vi "comm_Write_ip.vi"() -> ()   [LabVIEW 2014]
panel:
  in  "Indicator":bool
  in  "stop":bool
  # "BOMET TEST COMUNICATION WRITE"
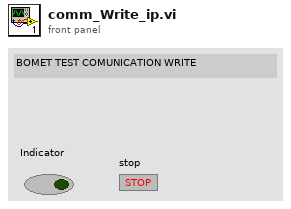
[diagram p1: front panel]
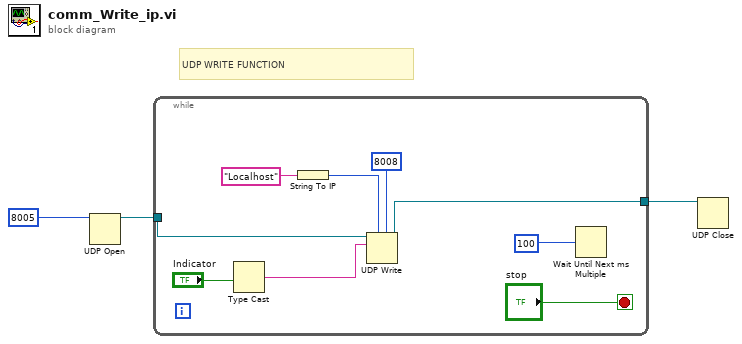
[diagram p0: block diagram]
diagram:
  # "UDP WRITE FUNCTION"
  n1 = UDP Open(11:u16 8005 ("port")) -> (port=w2:refnum<k16>)  [unwired: 4 in, 2 out]
  n2 = while {
    tunnel: w2 -> [w12]
    tunnel: [w11] -> w1
    stop <- "stop" stop-if-true
    n3 = Type Cast(x="Indicator") -> (*(type *) &x=w6:string)  [unwired: 1 in]
    n4 = String To IP(1:"Localhost" ("name")) -> (0:w9:u32)
    n5 = UDP Write(address=w9, port or service name=u16 8008, connection ID=w12, data in=w6) -> (3:w11:refnum<k16>)  [unwired: 2 in, 1 out]
    n6 = Wait Until Next ms Multiple(millisecond multiple=u32 100) -> ()  [unwired: 1 out]
  }
  n7 = UDP Close(connection ID=w1) -> ()  [unwired: 1 in, 2 out]
